vi "Periodic Tasks - Copy.vi"(3 "error in (no error)":errorcluster) -> ()   [LabVIEW 2011]
doc: "This VI runs in parallel to other tasks. It can contain as many user-defined periodic loops as you need. These can carry out PID or other sorts of timed response."
uses:
  <vilib>/Rock Robotics/SystemInterfaces/Utilities/FPGA_UtilitiesLED State.ctl
  <vilib>/Rock Robotics/SystemInterfaces/Utilities/FPGA_UtilitiesLED Source.ctl
  Robot Global Data.vi
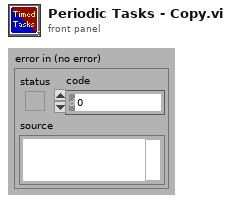
[diagram p1: front panel]
types:
  T1 = typedef "WPI_GyroDevRef.ctl" = cluster{"DevStatus":errorcluster, "Analog Module":T2, "Analog Channel":T3, "Offset":dbl, "Gain (VoltsPerDegree/Second)":dbl}
  T2 = typedef "FPGA_TypedefAnalogModule.ctl" = enum16{"Analog Module 1", "Analog Module 2"}
  T3 = typedef "FPGA_AIChannel.ctl" = enum8{"AI 1", "AI 2", "AI 3", "AI 4", "AI 5", "AI 6", "AI 7", "AI 8", "Invalid"}
  T4 = typedef "WPI_EncoderDevRef.ctl" = cluster{"DevStatus":errorcluster, "EncoderIndex":T5, "CounterIndex":T6, "DistancePerCount":dbl, "Decoding Type":T7}
  T5 = typedef "FPGA_EncoderIdx.ctl" = enum8{"Enc 0", "Enc 1", "Enc 2", "Enc 3", "Invalid"}
  T6 = typedef "FPGA_CounterCtrSystemIndex.ctl" = enum8{"Ctr 0", "Ctr 1", "Ctr 2", "Ctr 3", "Ctr 4", "Ctr 5", "Ctr 6", "Ctr 7", "Invalid"}
  T7 = typedef "WPI_EncoderType.ctl" = enum16{"1x", "2x", "4x"}
  T8 = typedef "FPGA_UtilitiesLED State.ctl" = enum16{"Off", "On", "Toggle"}
  T9 = typedef "FPGA_UtilitiesLED Source.ctl" = enum16{"User LED", "FPGA LED"}
  T10 = typedef "WPI_CompressorDevRef.ctl" = cluster{"DevStatus":errorcluster, "DigitalInputDevRef":T11, "RelayDevRef":T14}
  T11 = typedef "WPI_DigitalInputDevRef.ctl" = cluster{"DevStatus":errorcluster, "DIO Channel":T12, "Digital Module":T13}
  T12 = typedef "FPGA_DIOChannel.ctl" = enum8{"DIO 1", "DIO 2", "DIO 3", "DIO 4", "DIO 5", "DIO 6", "DIO 7", "DIO 8", "DIO 9", "DIO 10", "DIO 11", "DIO 12", "DIO 13", "DIO 14", "Invalid"}
  T13 = typedef "FPGA_TypedefDigitalModule.ctl" = enum16{"Digital Module 1", "Digital Module 2"}
  T14 = typedef "WPI_RelayDevRef.ctl" = cluster{"DevStatus":errorcluster, "Relay Channel":T15, "Digital Module":T13, "Relay Direction":T16}
  T15 = typedef "FPGA_DIORelayChannel.ctl" = enum8{"Relay 1", "Relay 2", "Relay 3", "Relay 4", "Relay 5", "Relay 6", "Relay 7", "Relay 8", "Invalid"}
  T16 = typedef "WPI_RelayDirection.ctl" = enum16{"Both directions", "Forward only", "Reverse only"}
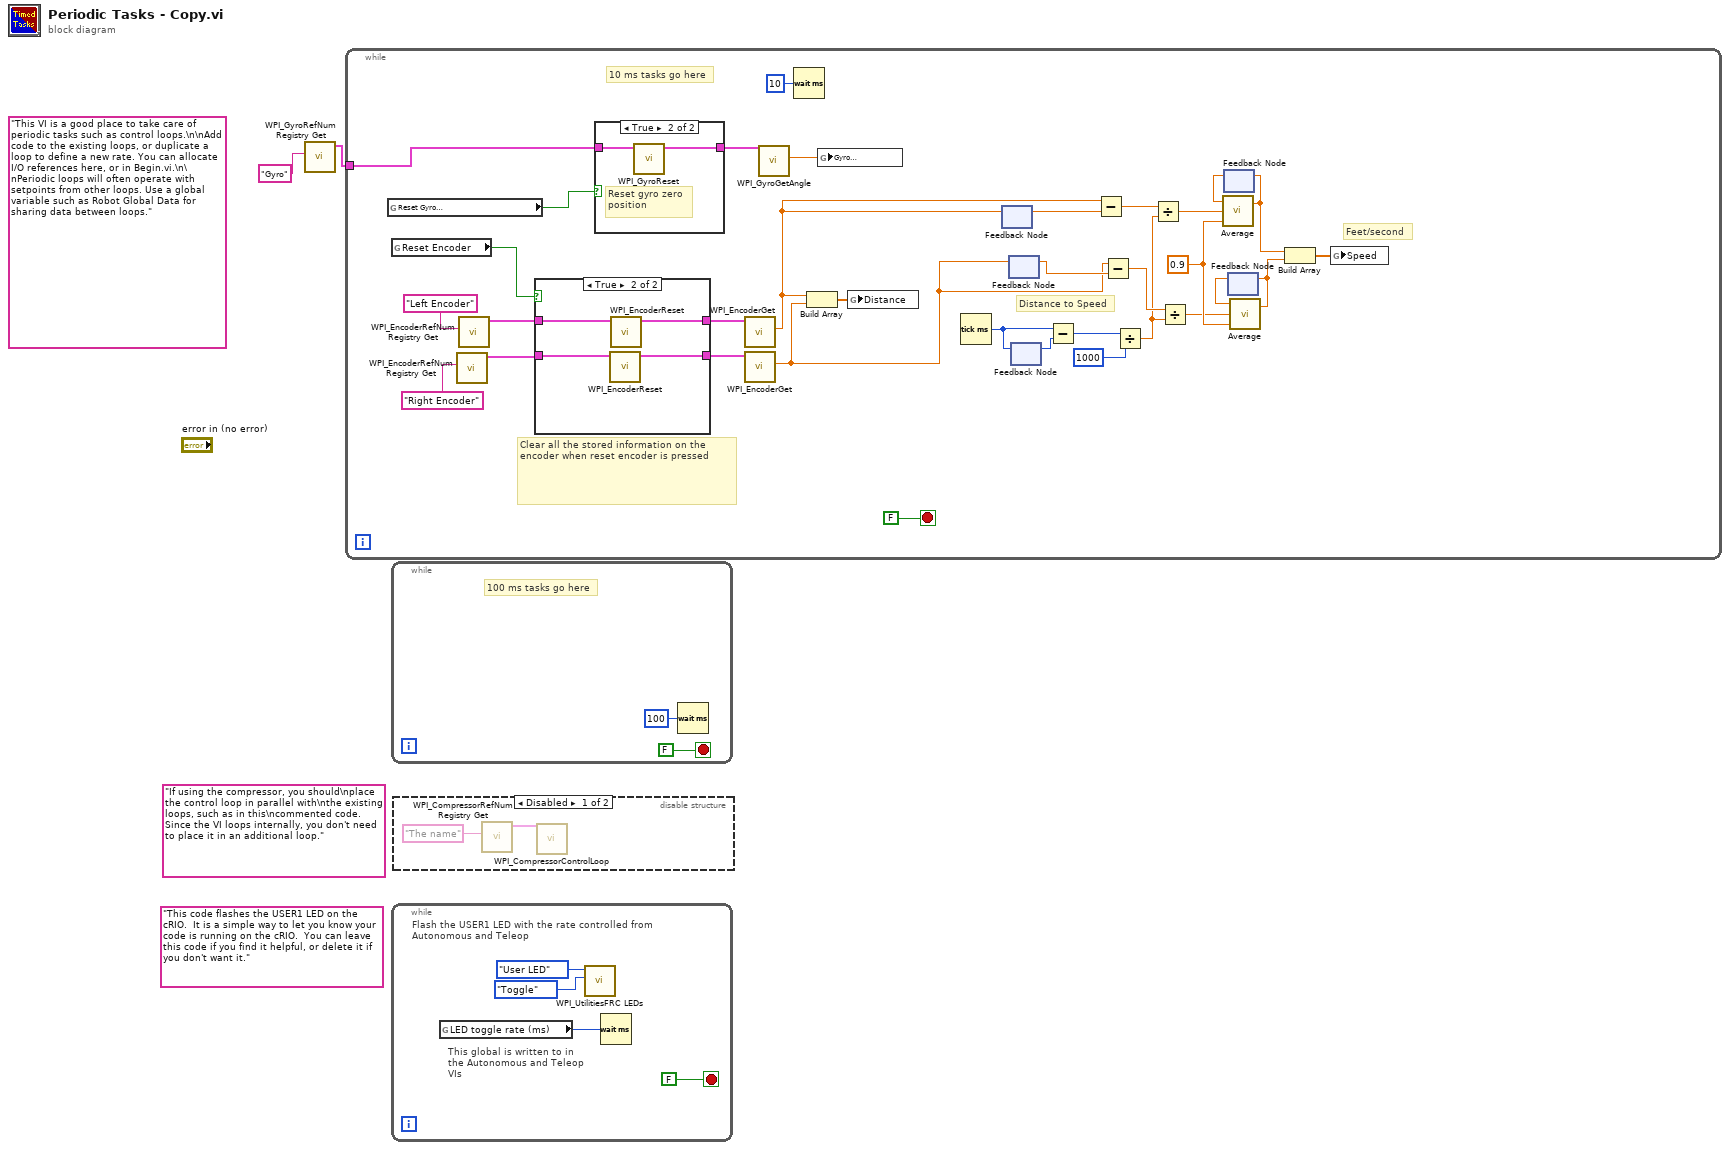
[diagram p0: block diagram]
diagram:
  (unwired) "If using the compressor, you should\nplace the control loop in parallel with\nthe existing loops, such as in this\ncommented code. Since the VI loops internally, you don't need to place it in an additional loop."
  (unwired) "This code flashes the USER1 LED on the cRIO.  It is a simple way to let you know your code is running on the cRIO.  You can leave this code if you find it helpful, or delete it if you don't want it."
  (unwired) "This VI is a good place to take care of periodic tasks such as control loops.\n\nAdd code to the existing loops, or duplicate a loop to define a new rate. You can allocate I/O references here, or in Begin.vi.\n\nPeriodic loops will often operate with setpoints from other loops. Use a global variable such as Robot Global Data for sharing data between loops."
  n1 = call <vilib>:"WPI_GyroRefNum Registry Get.vi"("refnum name"="Gyro") -> ("GyroDevRef"=w2:T1)  [unwired: 9 in, 1 out]
  n2 = while {
    tunnel: w2 -> [w22]
    stop <- FALSE stop-if-true
    w11 = 0.9 ("Speed avg. #")
    # "Feet/second"
    # "Distance to Speed"
    # "Clear all the stored information on the encoder when reset encoder is pressed"
    # "10 ms tasks go here"
    n3 = global read "Robot Global Data.vi" "Reset Gyro\nZero Position"() -> (w31:bool)
    n4 = global read "Robot Global Data.vi" "Reset Encoder"() -> (w23:bool)
    n5 = call <vilib>:"WPI_EncoderRefNum Registry Get.vi"("refnum name"="Right Encoder") -> ("EncoderDevRef"=w25:T4)  [unwired: 9 in, 1 out]
    n6 = call <vilib>:"WPI_EncoderRefNum Registry Get.vi"("refnum name"="Left Encoder") -> ("EncoderDevRef"=w28:T4)  [unwired: 9 in, 1 out]
    n7 = case shown="True" w23 {
      tunnel: w28 -> [w37 w41]
      tunnel: [w37 w40] -> w30
      tunnel: w25 -> [w36 w39]
      tunnel: [w36 w38] -> w29
      frame False {
      }
      frame True {
        n8 = call <vilib>:"WPI_EncoderReset.vi"("EncoderDevRef"=w39) -> ("EncoderDevRef"=w38:T4)  [unwired: 1 in, 9 out]
        n9 = call <vilib>:"WPI_EncoderReset.vi"("EncoderDevRef"=w41) -> ("EncoderDevRef"=w40:T4)  [unwired: 1 in, 9 out]
      }
    }
    n10 = case shown="True" w31 {
      tunnel: w22 -> [w42 w44]
      tunnel: [w42 w43] -> w33
      frame False {
      }
      frame True {
        # "Reset gyro zero \nposition"
        n11 = call <vilib>:"WPI_GyroReset.vi"("GyroDevRef"=w44) -> ("GyroDevRef"=w43:T1)  [unwired: 10 out]
      }
    }
    n12 = call <vilib>:"WPI_EncoderGet.vi"("EncoderDevRef"=w30) -> ("Distance"=w5:dbl)  [unwired: 1 in, 9 out]
    n13 = call <vilib>:"WPI_EncoderGet.vi"("EncoderDevRef"=w29) -> ("Distance"=w4:dbl)  [unwired: 1 in, 9 out]
    n14 = call <vilib>:"WPI_GyroGetAngle.vi"("GyroDevRef"=w33) -> ("Angle"=w32:dbl)  [unwired: 1 in, 9 out]
    n15 = Wait (ms)(milliseconds to wait=u32 10) -> ()  [unwired: 1 out]
    n16 = Build Array(w5, w4) -> (w24:dbl[])
    n17 = global write "Robot Global Data.vi" "Gyro\nAngle"(w32) -> ()
    n18 = global write "Robot Global Data.vi" "Distance"(w24) -> ()
    n19 = Tick Count (ms)() -> (millisecond timer value=w20:u32)
    n20 = feedback #1() -> (w19:dbl)  [unwired: 1 in]
    n21 = feedback-in #1(w5) -> ()
    n22 = feedback #2() -> (w14:dbl)  [unwired: 1 in]
    n23 = feedback-in #2(w4) -> ()
    n24 = feedback #3() -> (w21:u32)  [unwired: 1 in]
    n25 = feedback-in #3(w20) -> ()
    n26 = Subtract(x=w20, y=w21) -> (x-y=w17:u32)
    n27 = Subtract(x=w5, y=w19) -> (x-y=w18:dbl)
    n28 = Subtract(x=w4, y=w14) -> (x-y=w15:dbl)
    n29 = Divide(x=w17, y=u32 1000) -> (x/y=w6:dbl)
    n30 = Divide(x=w18, y=w6) -> (x/y=w9:dbl)
    n31 = Divide(x=w15, y=w6) -> (x/y=w10:dbl)
    n32 = feedback #4() -> (w12:dbl)  [unwired: 1 in]
    n33 = call "Average.vi"("averg #"=w11, "Input"=w9, "Previous\nValue"=w12) -> ("Output"=w8:dbl)  [unwired: 1 in]
    n34 = feedback-in #4(w8) -> ()
    n35 = feedback #5() -> (w13:dbl)  [unwired: 1 in]
    n36 = call "Average.vi"("averg #"=w11, "Input"=w10, "Previous\nValue"=w13) -> ("Output"=w7:dbl)  [unwired: 1 in]
    n37 = feedback-in #5(w7) -> ()
    n38 = Build Array(w8, w7) -> (w3:dbl[])
    n39 = global write "Robot Global Data.vi" "Speed"(w3) -> ()
  }
  n40 = while {
    stop <- FALSE stop-if-true
    # "100 ms tasks go here"
    n41 = Wait (ms)(milliseconds to wait=u32 100) -> ()  [unwired: 1 out]
  }
  n42 = while {
    stop <- FALSE stop-if-true
    # "This global is written to in the Autonomous and Teleop VIs"
    # "Flash the USER1 LED with the rate controlled from Autonomous and Teleop"
    n43 = global read "Robot Global Data.vi" "LED toggle rate (ms)"() -> (w47:u32)
    n44 = call <vilib>:"WPI_UtilitiesFRC LEDs.vi"("State"=FPGA_UtilitiesLED_State."Toggle", "LED Type"=FPGA_UtilitiesLED_Source."User LED") -> ()  [unwired: 1 in, 9 out]
    n45 = Wait (ms)(milliseconds to wait=w47) -> ()  [unwired: 1 out]
  }
  n46 = disable-structure shown="Disabled" {
    frame Disabled {
      n47 = call <vilib>:"WPI_CompressorRefNum Registry Get.vi"("refnum name"="The name") -> ("CompressorDevRef"=w52:T10)  [unwired: 9 in, 1 out]
      n48 = call <vilib>:"WPI_CompressorControlLoop.vi"("CompressorDevRef"=w52) -> ()  [unwired: 11 in]
    }
    frame Enabled {
    }
  }
